vi "Config ARB High Crest Mode.vi"(0 "VISA Resource Name":refnum<visa-resource-name>, 5 "State (F: OFF)":bool, 11 "error in (no error)":errorcluster {"code" format="%.0x"}) -> (4 "VISA Resource Name Out":refnum<visa-resource-name>, 15 "error out":errorcluster {"code" format="%.0x"})   [LabVIEW 2012, in "Agilent ESG Series.lvlib"]
doc: "This VI enables or disables the operating state of the high crest mode.\n\nNotes:\n(1) This VI is valid only on instrument E4438C with options 001/601 or 002/602."
uses:
  <instrlib>/Agilent ESG Series/Agilent ESG Series.lvlib
panel:
  # "ON"
  # "OFF"
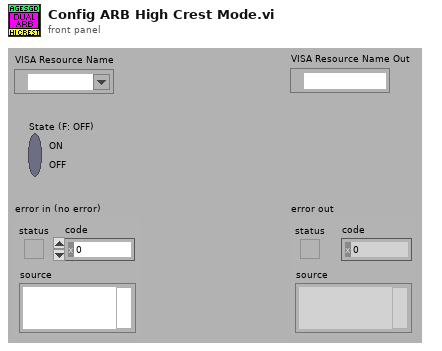
[diagram p1: front panel]
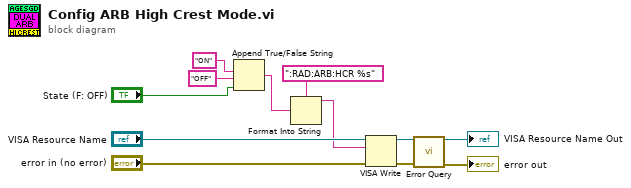
[diagram p0: block diagram]
diagram:
  n1 = Append True/False String(1:"State (F: OFF)", 2:"OFF" ("false string"), 3:"ON" ("multi-line string")) -> (0:w4:string)  [unwired: 1 in]
  n2 = Format Into String(format string=":RAD:ARB:HCR %s", w4) -> (resulting string=w3:string)  [unwired: 2 in, 1 out]
  n3 = VISA Write(VISA resource name="VISA Resource Name", write buffer=w3, error in (no error)="error in (no error)") -> (VISA resource name out=w8:refnum<visa-resource-name>, error out=w7:errorcluster)  [unwired: 1 out]
  n4 = call <instrlib>:"Error Query.vi"("VISA Resource Name"=w8, "error in (no error)"=w7) -> ("VISA Resource Name Out"=→"VISA Resource Name Out":refnum<visa-resource-name>, "error out"=→"error out":errorcluster)  [unwired: 10 in, 2 out]
